vi "Agilent 364xA (GPIB,Serial) Main Page.vi"(8 "error in (no error)":errorcluster, 11 "Node Ptr":T1 format="%.0x") -> (0 "error out":errorcluster)   [LabVIEW 2010, in "Agilent 364xA (GPIB,Serial) Custom Device.lvlib"]
uses:
  Agilent 364xA (GPIB,Serial) Custom Device.lvlib
  <vilib>/NI VeriStand/Custom Device API/Custom Device Item Ref.ctl
  Global Strings.vi
  <vilib>/NI VeriStand/Custom Device API/Get Item Property (Boolean).vi
  <vilib>/NI VeriStand/Custom Device API/Get Item Property (Double).vi
  <vilib>/NI VeriStand/Custom Device API/Get Item Property (String).vi
  <vilib>/NI VeriStand/Custom Device API/Get Item Property (U16).vi
  <vilib>/NI VeriStand/Custom Device API/Set Item Property (String).vi
  <vilib>/NI VeriStand/Custom Device API/Set Item Property (Boolean).vi
  <vilib>/NI VeriStand/Custom Device API/Set Item Property (Double).vi
  <vilib>/NI VeriStand/Custom Device API/Set Item Property (U16).vi
  <vilib>/NI Veristand/Custom Device API/Custom Device API.lvlib
panel:
  in  "Perform ID Query?":bool=TRUE
  in  "Loop rate (ms)":u16
  in  "Voltage Limit":dbl(slide)=20.0 min=1.0 max=60.0 scale=1.0..36.0 scale format="%#.6g"
  in  "Enable OVP":bool=TRUE
  in  "VISA resource name":string
  in  "Header":cluster{"Section Name":string}={"Section Name"="Agilent 364xA Item Settings"}
  in  "Description":string
  in  "Name":string
  in  "Delete":bool
  # "If you're using a serial interface: Configure the serial interface in Devices & Interfaces -> Ports -> Com# in Measurement and Automation Explorer"
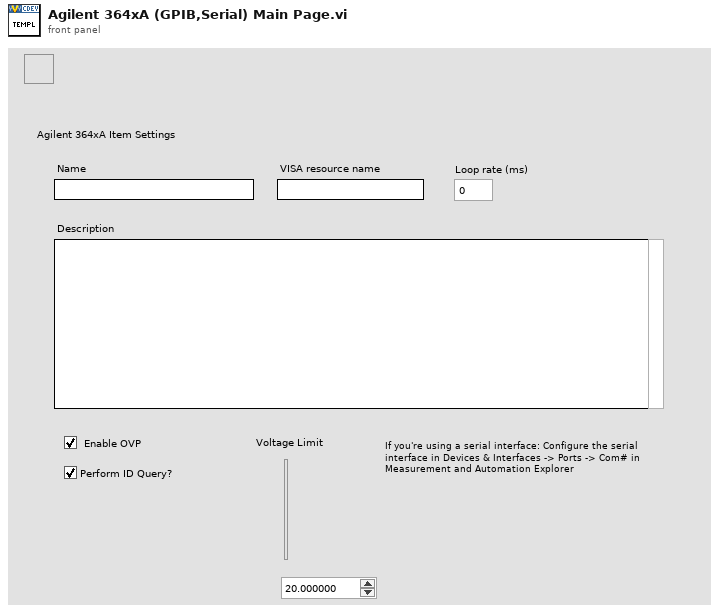
[diagram p1: front panel]
types:
  T1 = typedef "Custom Device API.lvlib/Custom Device Item Ref.ctl" = u64
  T2 = typedef "Custom Device API.lvlib/Custom Device Item Info.ctl" = cluster{"Name":string, "Is Channel":bool, "GUID":string}
  T3 = typedef "Custom Device API.lvlib/Custom Device Commands.ctl" = enum16{"Default", "Item renamed", "Shutdown", "Dynamic button pressed"}
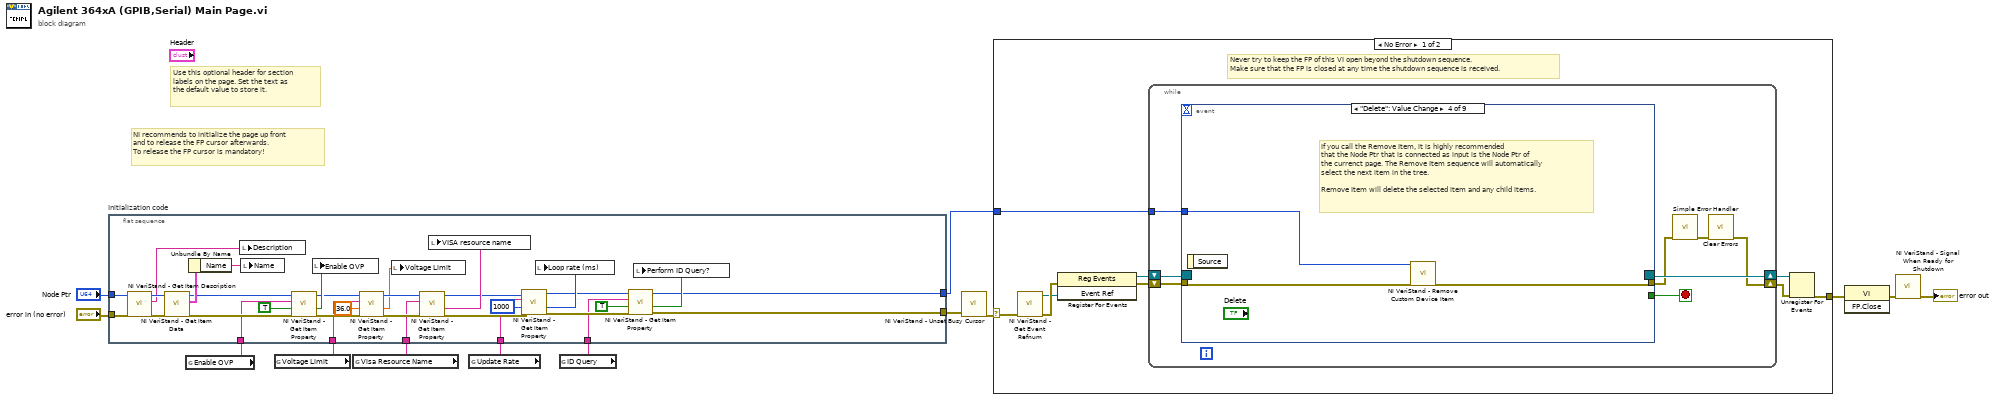
[diagram p0: block diagram]
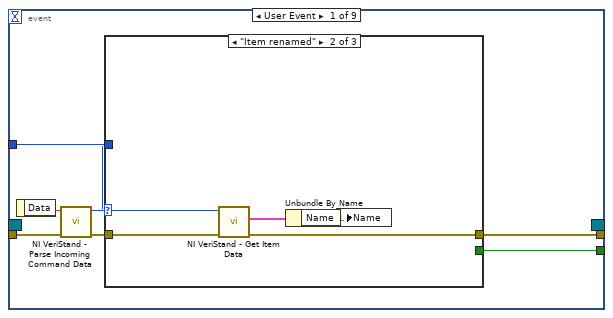
[diagram p2: hidden frame]
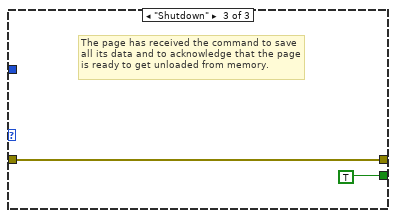
[diagram p4: hidden frame]
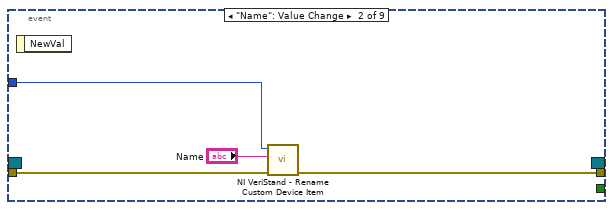
[diagram p5: hidden frame]
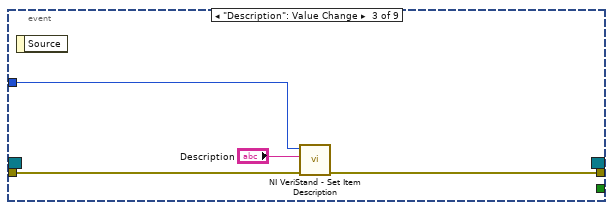
[diagram p6: hidden frame]
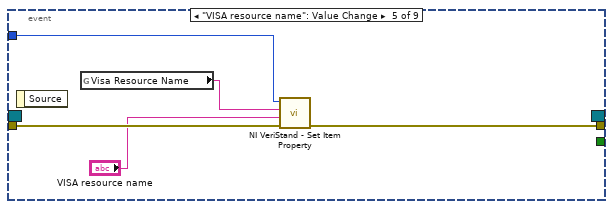
[diagram p7: hidden frame]
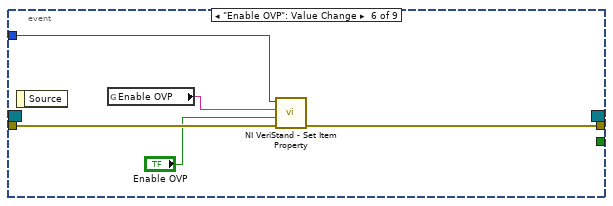
[diagram p8: hidden frame]
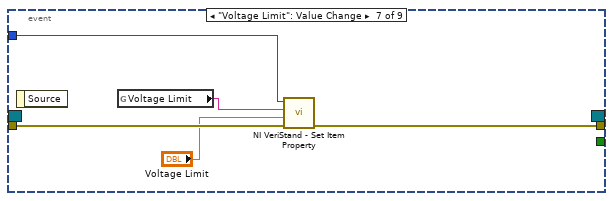
[diagram p9: hidden frame]
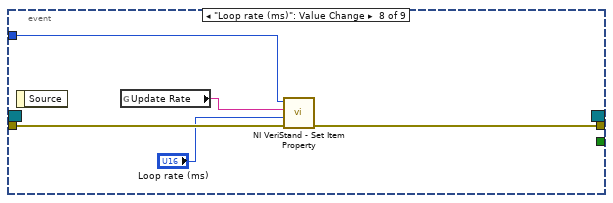
[diagram p10: hidden frame]
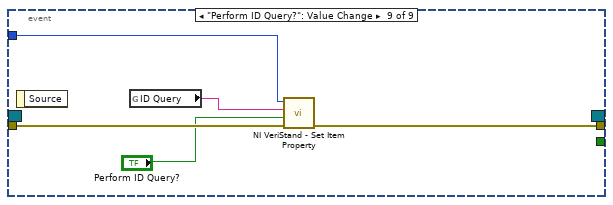
[diagram p11: hidden frame]
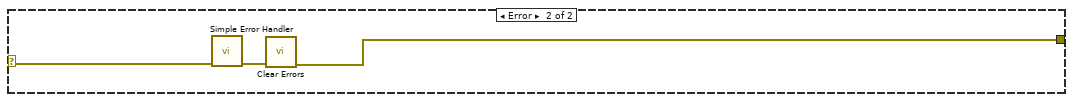
[diagram p12: hidden frame]
diagram:
  # "Use this optional header for section labels on the page. Set the text as the default value to store it."
  # "NI recommends to initialize the page up front\nand to release the FP cursor afterwards.\nTo release the FP cursor is mandatory!"
  n1 = flat-sequence "Initialization code" {
    tunnel: "error in (no error)" -> [w45]
    tunnel: "Node Ptr" -> [w44]
    tunnel: [w14] -> w7
    tunnel: w6 -> [w37]
    tunnel: w5 -> [w32]
    tunnel: w4 -> [w28]
    tunnel: w3 -> [w24]
    tunnel: w2 -> [w18]
    tunnel: [w15] -> w1
    frame #0 {
      n2 = call <vilib>:"NI VeriStand - Get Item Description.vi"("error in (no error)"=w45, "Item Ref in"=w44) -> ("error out"=w42:errorcluster, "Description"=w43:string, "Item Ref out"=w46:T1)  [unwired: 7 out]
      n3 = call <vilib>:"NI VeriStand - Get Item Data.vi"("error in (no error)"=w42, "Item Ref in"=w46) -> ("error out"=w39:errorcluster, "Item Info"=w41:T2, "Item Ref out"=w38:T1)  [unwired: 7 out]
      n4 = Unbundle By Name(w41) -> ("Name"=w40:string)
      n5 = local write "Description"(w43) -> ()
      n6 = local write "Name"(w40) -> ()
      n7 = call-poly <vilib>:"NI VeriStand - Get Item Property.vi"("error in (no error)"=w39, "Default Value"=TRUE, "Property Name"=w37, "Item Ref in"=w38) -> ("error out"=w34:errorcluster, "Value"=w35:bool, "Item Ref out"=w33:T1)  [unwired: 4 in, 1 out]
      n8 = local write "Enable OVP"(w35) -> ()
      n9 = call-poly <vilib>:"NI VeriStand - Get Item Property.vi"("error in (no error)"=w34, "Default Value"=36.0, "Property Name"=w32, "Item Ref in"=w33) -> ("error out"=w30:errorcluster, "Value"=w27:dbl, "Item Ref out"=w29:T1)  [unwired: 4 in, 1 out]
      n10 = local write "Voltage Limit"(w27) -> ()
      n11 = call-poly <vilib>:"NI VeriStand - Get Item Property.vi"("error in (no error)"=w30, "Property Name"=w28, "Item Ref in"=w29) -> ("error out"=w25:errorcluster, "Value"=w26:string, "Item Ref out"=w23:T1)  [unwired: 5 in, 1 out]
      n12 = local write "VISA resource name"(w26) -> ()
      n13 = call-poly <vilib>:"NI VeriStand - Get Item Property.vi"("error in (no error)"=w25, "Default Value"=u16 1000, "Property Name"=w24, "Item Ref in"=w23) -> ("error out"=w20:errorcluster, "Value"=w21:u16, "Item Ref out"=w19:T1)  [unwired: 4 in, 1 out]
      n14 = local write "Loop rate (ms)"(w21) -> ()
      n15 = call-poly <vilib>:"NI VeriStand - Get Item Property.vi"("error in (no error)"=w20, "Default Value"=TRUE, "Property Name"=w18, "Item Ref in"=w19) -> ("error out"=w15:errorcluster, "Value"=w16:bool, "Item Ref out"=w14:T1)  [unwired: 4 in, 1 out]
      n16 = local write "Perform ID Query?"(w16) -> ()
    }
  }
  n17 = global read "Global Strings.vi" "Enable OVP"() -> (w6:string)
  n18 = global read "Global Strings.vi" "Voltage Limit"() -> (w5:string)
  n19 = global read "Global Strings.vi" "Visa Resource Name"() -> (w4:string)
  n20 = global read "Global Strings.vi" "Update Rate"() -> (w3:string)
  n21 = global read "Global Strings.vi" "ID Query"() -> (w2:string)
  n22 = call <vilib>:"NI VeriStand - Unset Busy Cursor.vi"("error in (no error)"=w1) -> ("error out"=w9:errorcluster)  [unwired: 10 out]
  n23 = case shown="No Error" w9 {
    selector: w9 -> [w47 w117]
    tunnel: [w52 w115] -> w13
    tunnel: w7 -> [w48 _]
    frame No Error {
      # "Never try to keep the FP of this VI open beyond the shutdown sequence.\nMake sure that the FP is closed at any time the shutdown sequence is received."
      n24 = call <vilib>:"NI VeriStand - Get Event Refnum.vi"("error in (no error)"=w47) -> ("error out"=w55:errorcluster, "Event Ref"=w51:refnum<user-event>)  [unwired: 9 out]
      n25 = register-events(error in=w55, w51) -> (reference out=w49:refnum<event-registration>, error out=w50:errorcluster)  [unwired: 1 in]
      n26 = while {
        tunnel: w48 -> [w59]
        shift-right: [w56] -> w53
        shift-left: w50 -> [w62]
        shift-right: [w63] -> w54
        shift-left: w49 -> [w61]
        stop <- w60 stop-if-true
        n27 = event shown="[3] \"Delete\": Value Change" {
          selector: w61 -> [_ _ _ _ _ _ _ _ _]
          dyn-events: [_ _ _ _ _ _ _ _ _] -> w63
          timeout: _ -> [_ _ _ _ _ _ _ _ _]
          tunnel: w62 -> [w70 w82 w85 w89 w94 w99 w104 w109 w114]
          tunnel: [w66 _ _ _ _ _ _ _ _] -> w60
          tunnel: [w65 w81 w84 w88 w93 w98 w103 w108 w113] -> w58
          tunnel: w59 -> [w64 w80 w86 w87 w92 w97 w100 w106 w111]
          event User Event {
            n28 = event-data() -> ("Data"=w69:string)  [unwired: 1 out]
            n29 = call <vilib>:"NI VeriStand - Parse Incoming Command Data.vi"("error in (no error)"=w70, "Data"=w69) -> ("error out"=w68:errorcluster, "Action"=w67:T3)  [unwired: 8 out]
            n30 = case shown="\"Item renamed\"" w67 {
              tunnel: w68 -> [w71 w76 w77]
              tunnel: [_ _ TRUE] -> w66
              tunnel: [w71 w73 w77] -> w65
              tunnel: w64 -> [_ w75 _]
              frame "Default", Default {
              }
              frame "Item renamed" {
                n31 = call <vilib>:"NI VeriStand - Get Item Data.vi"("error in (no error)"=w76, "Item Ref in"=w75) -> ("error out"=w73:errorcluster, "Item Info"=w74:T2)  [unwired: 8 out]
                n32 = Unbundle By Name(w74) -> ("Name"=w72:string)
                n33 = local write "Name"(w72) -> ()
              }
              frame "Shutdown" {
                # "The page has received the command to save all its data and to acknowledge that the page is ready to get unloaded from memory."
              }
            }
          }
          event "Name": Value Change {
            n34 = event-data() -> ()  [unwired: 2 out]
            n35 = call <vilib>:"NI VeriStand - Rename Custom Device Item.vi"("error in (no error)"=w82, "New Name"="Name", "Item Ref in"=w80) -> ("error out"=w81:errorcluster)  [unwired: 8 out]
          }
          event "Description": Value Change {
            n36 = event-data() -> ()  [unwired: 2 out]
            n37 = call <vilib>:"NI VeriStand - Set Item Description.vi"("error in (no error)"=w85, "Description"="Description", "Item Ref in"=w86) -> ("error out"=w84:errorcluster)  [unwired: 8 out]
          }
          event "Delete": Value Change {
            # "If you call the Remove Item, it is highly recommended\nthat the Node Ptr that is connected as input is the Node Ptr of\nthe currenct page. The Remove Item sequence will automatically\nselect the next item in the tree.\n\nRemove Item will delete the selected item and any child items."
            n38 = event-data() -> ()  [unwired: 2 out]
            n39 = call <vilib>:"NI VeriStand - Remove Custom Device Item.vi"("error in (no error)"=w89, "Item Ref in"=w87) -> ("error out"=w88:errorcluster)  [unwired: 1 in, 8 out]
          }
          event "VISA resource name": Value Change {
            n40 = event-data() -> ()  [unwired: 2 out]
            n41 = global read "Global Strings.vi" "Visa Resource Name"() -> (w91:string)
            n42 = call-poly <vilib>:"NI VeriStand - Set Item Property.vi"("error in (no error)"=w94, "Value"="VISA resource name", "Property Name"=w91, "Item Ref in"=w92) -> ("error out"=w93:errorcluster)  [unwired: 5 in, 2 out]
          }
          event "Enable OVP": Value Change {
            n43 = event-data() -> ()  [unwired: 2 out]
            n44 = global read "Global Strings.vi" "Enable OVP"() -> (w96:string)
            n45 = call-poly <vilib>:"NI VeriStand - Set Item Property.vi"("error in (no error)"=w99, "Value"="Enable OVP", "Property Name"=w96, "Item Ref in"=w97) -> ("error out"=w98:errorcluster)  [unwired: 5 in, 2 out]
          }
          event "Voltage Limit": Value Change {
            n46 = event-data() -> ()  [unwired: 2 out]
            n47 = global read "Global Strings.vi" "Voltage Limit"() -> (w101:string)
            n48 = call-poly <vilib>:"NI VeriStand - Set Item Property.vi"("error in (no error)"=w104, "Value"="Voltage Limit", "Property Name"=w101, "Item Ref in"=w100) -> ("error out"=w103:errorcluster)  [unwired: 5 in, 2 out]
          }
          event "Loop rate (ms)": Value Change {
            n49 = event-data() -> ()  [unwired: 2 out]
            n50 = global read "Global Strings.vi" "Update Rate"() -> (w107:string)
            n51 = call-poly <vilib>:"NI VeriStand - Set Item Property.vi"("error in (no error)"=w109, "Value"="Loop rate (ms)", "Property Name"=w107, "Item Ref in"=w106) -> ("error out"=w108:errorcluster)  [unwired: 5 in, 2 out]
          }
          event "Perform ID Query?": Value Change {
            n52 = event-data() -> ()  [unwired: 2 out]
            n53 = global read "Global Strings.vi" "ID Query"() -> (w112:string)
            n54 = call-poly <vilib>:"NI VeriStand - Set Item Property.vi"("error in (no error)"=w114, "Value"="Perform ID Query?", "Property Name"=w112, "Item Ref in"=w111) -> ("error out"=w113:errorcluster)  [unwired: 5 in, 2 out]
          }
        }
        n55 = call <vilib>:"Simple Error Handler.vi"("error in (no error)"=w58) -> ("error out"=w57:errorcluster)  [unwired: 1 in, 7 out]
        n56 = call <vilib>:"Clear Errors.vi"("error in (no error)"=w57) -> ("error out"=w56:errorcluster)  [unwired: 6 out]
      }
      n57 = Unregister For Events(event registration refnum=w54, error in=w53) -> (error out=w52:errorcluster)
    }
    frame Error {
      n58 = call <vilib>:"Simple Error Handler.vi"("error in (no error)"=w117) -> ("error out"=w116:errorcluster)  [unwired: 1 in, 7 out]
      n59 = call <vilib>:"Clear Errors.vi"("error in (no error)"=w116) -> ("error out"=w115:errorcluster)  [unwired: 6 out]
    }
  }
  n60 = invoke class="VI" method="FP.Close"(error in=w13) -> (error out=w12:errorcluster)  [unwired: 2 in, 2 out]
  n61 = call <vilib>:"NI VeriStand - Signal When Ready for Shutdown.vi"("error in (no error)"=w12) -> ("error out"=→"error out":errorcluster)  [unwired: 10 out]
